vi "S2C_ExeTableFGV.vi"(7 "Action":enum16{"Get", "Set"}(ring), 8 "Error In":errorcluster, 11 "Table In":string[][](array[string])) -> (0 "Error Out":errorcluster, 3 "Table Out":string[][](array[string]))   [LabVIEW 2015]
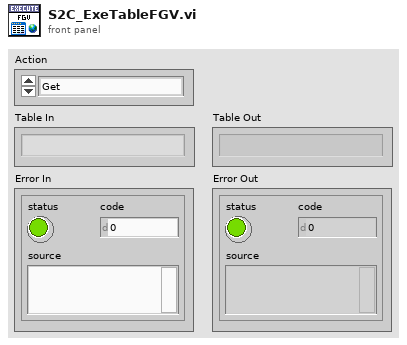
[diagram p1: front panel]
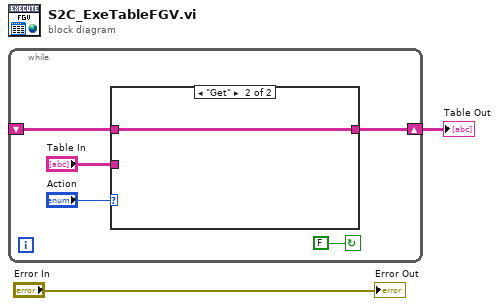
[diagram p0: block diagram]
diagram:
  n1 = while {
    shift-right: [w5] -> w1
    shift-left: _ -> [w4]
    stop <- FALSE continue-if-true
    n2 = case shown="\"Get\"" "Action" {
      tunnel: [w8 w9] -> w5
      tunnel: w4 -> [_ w9]
      tunnel: "Table In" -> [w8 _]
      frame "Set" {
      }
      frame "Get" {
      }
    }
  }
  "Table Out" <- w1
  "Error Out" <- "Error In"
